vi "find middle delay.vi"(1 "array of times":dbl[unit][](array[numeric]), 2 "Expected overall period":dbl[unit]) -> (0 "middle delay":dbl[unit])   [LabVIEW 2015]
doc: "\"middle delay\" = T/2 - (sum of most of the other times in time array)\n \"most of the other elements\": \n if even number of elements in time array, go from 2 to N\n if odd number of elements in time array, go from 2 to N-1"
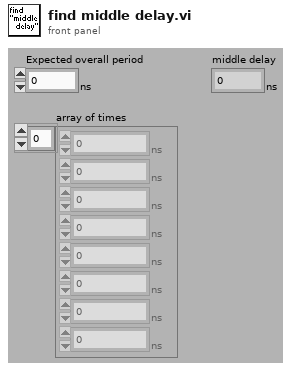
[diagram p1: front panel]
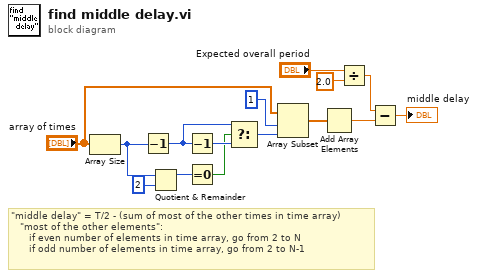
[diagram p0: block diagram]
diagram:
  # "\"middle delay\" = T/2 - (sum of most of the other times in time array)\n   \"most of the other elements\": \n      if even number of elements in time array, go from 2 to N\n      if odd number of elements in time array, go from 2 to N-1"
  n1 = Array Size(array="array of times") -> (size(s)=w7:i32)
  n2 = Decrement(x=w7) -> (x-1=w9:i32)
  n3 = Quotient & Remainder(x=w7, y=i8 2) -> (x-y*floor(x/y)=w6:i32)  [unwired: 1 out]
  n4 = Decrement(x=w9) -> (x-1=w8:i32)
  n5 = Equal To 0?(x=w6) -> (x = 0?=w5:bool)
  n6 = Select(t=w9, s=w5, f=w8) -> (s? t:f=w11:i32)
  n7 = Array Subset(array="array of times", index=1, length=w11) -> (w12:dbl[unit][])
  n8 = Add Array Elements(numeric array=w12) -> (sum=w14:dbl[unit])
  n9 = Divide(x="Expected overall period", y=2.0) -> (x/y=w2:dbl[unit])
  n10 = Subtract(x=w2, y=w14) -> (x-y=→"middle delay":dbl[unit])
